vi "UTIL Get Session Prefix.vi"(7 "Session - Root":refnum<class "niRFUtil Session.lvclass">) -> (8 "Session Prefix":string)   [LabVIEW 2016, in "niRFUtil.lvlib" / "niRFUtil Session.lvclass"]
doc: "Obtain the prefix for the session to prevent name collisions.\n\nRoot class has its own prefix, but child classes should append their own to ensure that two different session types can have the same name."
uses:
  niRFUtil Session.lvclass
  niRFUtil Session.lvclass/niRFUtil Session.ctl
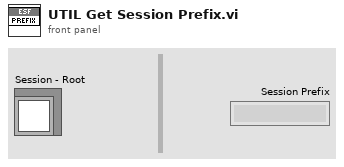
[diagram p1: front panel]
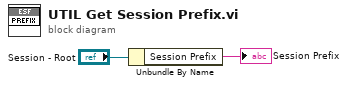
[diagram p0: block diagram]
diagram:
  n1 = Unbundle By Name("Session - Root") -> ("Session Prefix"=→"Session Prefix":string)
